vi "Initialize MeasurementLink Session.vi"(7 "remote connection options":T2, 8 "error in":errorcluster, 9 "initialize and close session behavior":T1, 10 "session initialization parameters":T3, 11 "session factory in":refnum<class "Session Factory.lvclass">) -> (0 "error out":errorcluster, 2 "session out":variant, 3 "session factory out":refnum<class "Session Factory.lvclass">)   [LabVIEW 2020, in "VISA Sessions.lvlib" / "Session Factory.lvclass"]
uses:
  Session Factory.lvclass
  Instrument Sessions/ISession Factory/Session Initialization Parameters.ctl
  Instrument Sessions/ISession Factory/Remote Connection Options.ctl
  Instrument Sessions/ISession Factory/Initialize and Close Session Behavior.ctl
  Session Factory.lvclass/Session Factory.ctl
  Instrument Sessions/ISession Factory/ISession Factory.lvclass
  <vilib>/NI-VISA/VISA Open for gRPC Session.vi
  To VISA Init and Close Enum.vi
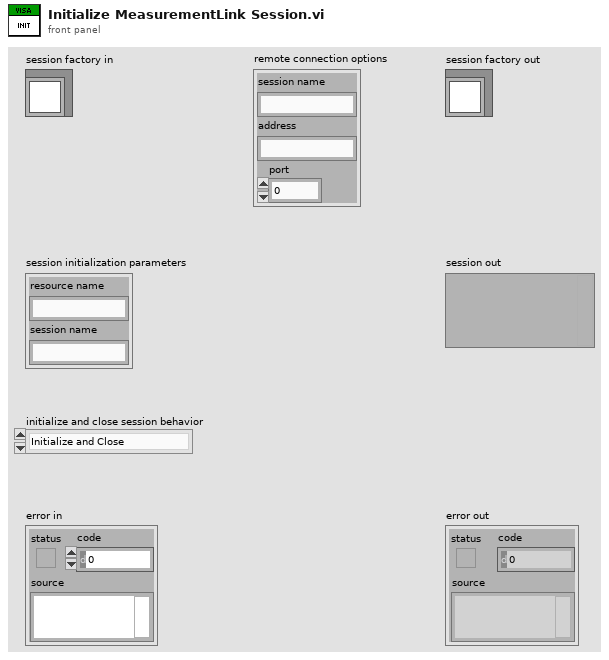
[diagram p1: front panel]
types:
  T1 = typedef "Instrument Sessions.lvlib/ISession Factory.lvclass/Initialize and Close Session Behavior.ctl" = enum16{"Initialize and Close", "Attach and Detach", "Initialize and Detach", "Attach and Close"}
  T2 = typedef "Instrument Sessions.lvlib/ISession Factory.lvclass/Remote Connection Options.ctl" = cluster{"session name":string, "address":string, "port":u32}
  T3 = typedef "Instrument Sessions.lvlib/ISession Factory.lvclass/Session Initialization Parameters.ctl" = cluster{"resource name":string, "session name":string}
  T4 = typedef "VISA Open Access Mode.ctl" = u32
  T5 = typedef "VISA gRPC Open Close Behavior.ctl" = enum16{"Auto", "Initialize and Close", "Attach and Detach", "Initialize and Detach", "Attach and Close"}
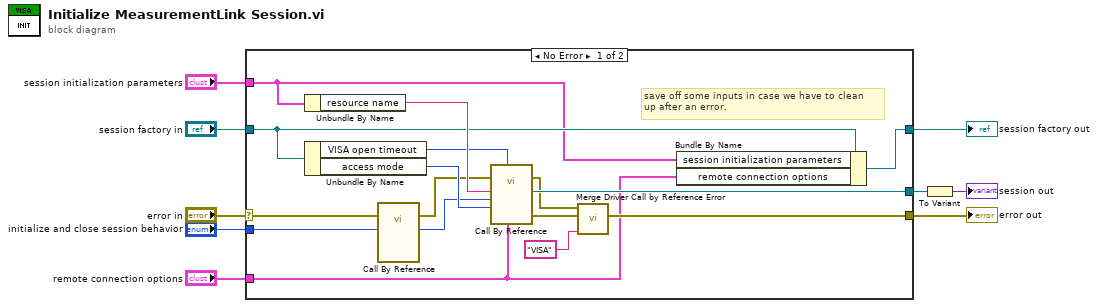
[diagram p0: block diagram]
diagram:
  n1 = case shown="No Error" "error in" {
    selector: "error in" -> [w15 w26]
    tunnel: [w21 w26] -> w8
    tunnel: "session factory in" -> [w13 w27]
    tunnel: [w12 w27] -> w6
    tunnel: "remote connection options" -> [w11 _]
    tunnel: "session initialization parameters" -> [w10 _]
    tunnel: [w25 _] -> w3
    tunnel: "initialize and close session behavior" -> [w17 _]
    frame No Error {
      # "save off some inputs in case we have to clean\nup after an error."
      n2 = Unbundle By Name(w10) -> ("resource name"=w24:string)
      n3 = Unbundle By Name(w13) -> ("VISA open timeout"=w18:u32, "access mode"=w19:T4)
      n4 = call-by-ref "?"(error in=w15, "factory init and close behavior"=w17) -> (error out=w14:errorcluster, "visa init and close behavior"=w16:T5)  [unwired: 11 in, 1 out]
      n5 = call-by-ref "?"(error in=w14, "gRPC Options"=w11, "VISA Open Timeout (0)"=w18, "Access Mode"=w19, "Open/Close Behavior"=w16, "VISA resource name"=w24) -> (error out=w22:errorcluster, 0:"error out"=w23:errorcluster, "VISA resource name out"=w25:refnum<visa-resource-name>)  [unwired: 6 in, 1 out]
      n6 = call "Merge Driver Call by Reference Error.vi"("driver name"="VISA", "called vi error"=w23, "call by ref error"=w22) -> ("error out"=w21:errorcluster)  [unwired: 8 in]
      n7 = Bundle By Name(cluster=w13, "session initialization parameters"=w10, "remote connection options"=w11) -> (w12:refnum<class "Session Factory.lvclass">)
    }
    frame Error {
    }
  }
  "error out" <- w8
  "session factory out" <- w6
  n8 = To Variant(anything=w3) -> (Variant=→"session out":variant)
